vi "Set GPU FFT Config.vi"(8 "error in (no error)":errorcluster, 9 "Batch Size":u64=100 format="%.0p FFT", 10 "FFT Size":u64=2000000 format="%.0p Samples", 11 "Application Manager in":refnum<class "Application Manager.lvclass">) -> (0 "error out":errorcluster, 3 "Application Manager out":refnum<class "Application Manager.lvclass">)   [LabVIEW 2020, in "Application Manager.lvlib" / "Application Manager.lvclass"]
uses:
  Application Manager.lvclass
  Application Manager.lvclass/Application Manager.ctl
  GPU FFT Calculator/GPU FFT Calculator Messages/Set FFT Config Msg/Set FFT Config Msg.lvclass/Set FFT Config Msg.ctl
  <vilib>/ActorFramework/Message Enqueuer/Message Enqueuer.lvclass/Message Enqueuer.ctl
  <vilib>/ActorFramework/Message Enqueuer/Enqueue.vi
  GPU FFT Calculator/GPU FFT Calculator Messages/Set FFT Config Msg/Set FFT Config Msg.lvclass
  C:/Program Files/National Instruments/LabVIEW 2026/vi.lib/ActorFramework/Message/Message.lvclass
  <vilib>/ActorFramework/Message Priority Queue/Priority Enqueue.vi
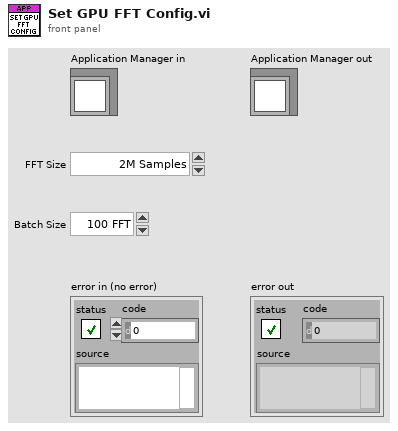
[diagram p1: front panel]
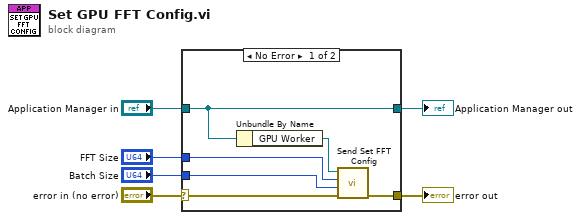
[diagram p0: block diagram]
diagram:
  n1 = case shown="No Error" "error in (no error)" {
    selector: "error in (no error)" -> [w10 w14]
    tunnel: [w9 w14] -> w5
    tunnel: [w12 w13] -> w3
    tunnel: "Application Manager in" -> [w12 w13]
    tunnel: "FFT Size" -> [w8 _]
    tunnel: "Batch Size" -> [w7 _]
    frame No Error {
      n2 = Unbundle By Name(w12) -> ("GPU Worker"=w11:refnum<class "Message Enqueuer.lvclass">)
      n3 = call "Send Set FFT Config.vi"("error in (no error)"=w10, "Batch Size"=w7, "FFT Size"=w8, "Message Enqueuer"=w11) -> ("error out"=w9:errorcluster)  [unwired: 6 in, 1 out]
    }
    frame Error {
    }
  }
  "error out" <- w5
  "Application Manager out" <- w3
